vi "Adresse Regler.vi"(8 "error in (no error)":errorcluster caption="Fehler (Eingang, kein Fehler)", 10 "Index":u16, 11 "Steuerung PNS Eingang":refnum<class "Steuerung PNS.lvclass">) -> (0 "error out":errorcluster caption="Fehler (Ausgang)", 2 "Adressen":T1, 3 "Steuerung PNS Ausgang":refnum<class "Steuerung PNS.lvclass">)   [LabVIEW 2020, in "Steuerung PNS.lvclass"]
uses:
  Steuerung PNS.lvclass
  Adresse.ctl
  AdressIndex.ctl
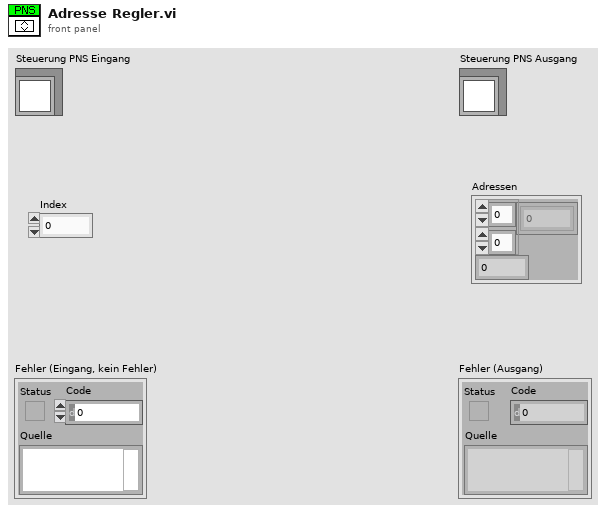
[diagram p1: front panel]
types:
  T1 = typedef "Steuerung PNS.lvclass/Adresse.ctl" = cluster{i32[][], i32}
  T2 = typedef "Steuerung PNS.lvclass/AdressIndex.ctl" = cluster{"Index":i32, "Index 2":i32, "Länge2":i32, "\nAnzahl":i32}
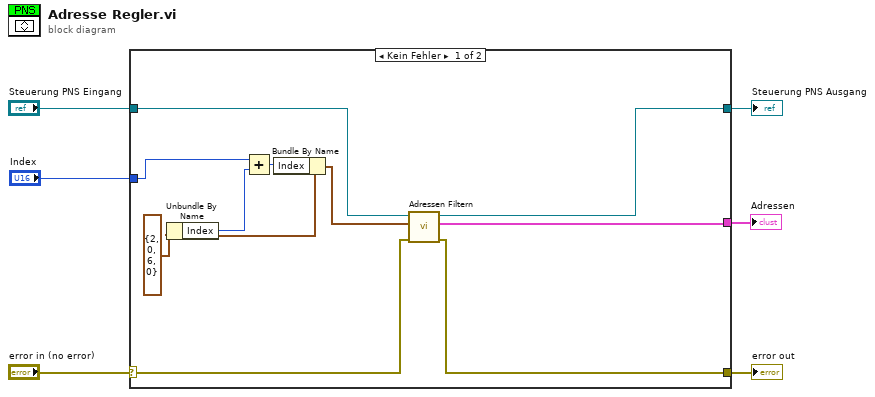
[diagram p0: block diagram]
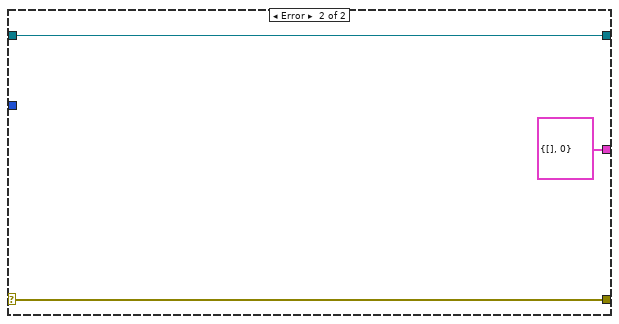
[diagram p2: hidden frame]
diagram:
  n1 = case shown="Kein Fehler" "error in (no error)" {
    selector: "error in (no error)" -> [w13 w19]
    tunnel: [w12 w19] -> w5
    tunnel: [w15 w18] -> w3
    tunnel: "Steuerung PNS Eingang" -> [w16 w18]
    tunnel: [w14 T1 {[], 0} ("Adressen")] -> w2
    tunnel: "Index" -> [w11 _]
    frame No Error {
      w8 = T2 {"Index"=2, "Index 2"=0, "Länge2"=6, "\nAnzahl"=0} ("AdressIndex")
      n2 = Unbundle By Name(w8) -> ("Index"=w10:i32)
      n3 = Add(x=w11, y=w10) -> (x+y=w9:i32)
      n4 = Bundle By Name(cluster=w8, "Index"=w9) -> (w7:T2)
      n5 = call "Adressen Filtern.vi"("error in (no error)"=w13, "AdressIndex"=w7, "Steuerung PNS Eingang"=w16) -> ("error out"=w12:errorcluster, "Adressen"=w14:cluster{i32[][], i32}, "Steuerung PNS Ausgang"=w15:refnum<class "Steuerung PNS.lvclass">)  [unwired: 6 in]
    }
    frame Error {
    }
  }
  "error out" <- w5
  "Steuerung PNS Ausgang" <- w3
  "Adressen" <- w2
